vi "AddTestSuite.vi"(8 "error in (no error)":errorcluster, 9 "Name":string, 10 "Parent Tag (\"\")":string, 11 "ResultTree in":refnum<class "ResultTree.lvclass">) -> (0 "error out":errorcluster, 2 "Tag Name":string, 3 "ResultTree out":refnum<class "ResultTree.lvclass">)   [LabVIEW 2017, in "ResultTree.lvclass"]
doc: "Adds a test suite. Returns the tag name.\n\nIf no parent tag is specified, the test suite is added to the root and tagged with the prefix \"SUITE_\" followed by the name of the suite.\n\nIf a parent tag is specified, the test suite is added as a child to the parent suite with the parent suite name as prefix followed by \"/\" and the name of the suite."
uses:
  ResultTree.lvclass
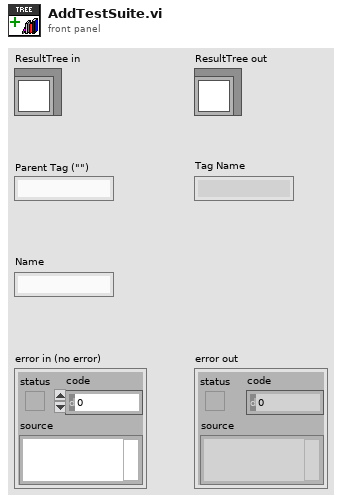
[diagram p1: front panel]
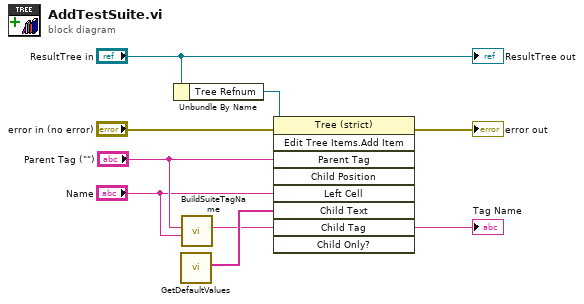
[diagram p0: block diagram]
diagram:
  n1 = Unbundle By Name("ResultTree in") -> ("Tree Refnum"=w5:refnum<vi>)
  n2 = call "GetDefaultValues.vi"() -> ("Default Values"=w4:string[])  [unwired: 11 in]
  n3 = call "BuildSuiteTagName.vi"("Suite Name"="Name", "Parent Tag"="Parent Tag (\"\")") -> ("Tag Name"=w1:string)  [unwired: 9 in]
  "Tag Name" <- w1
  n4 = invoke class="Tree (strict)" method="Edit Tree Items.Add Item"(reference=w5, error in="error in (no error)", "Parent Tag"="Parent Tag (\"\")", "Left Cell"="Name", "Child Text"=w4, "Child Tag"=w1) -> (error out=→"error out":errorcluster)  [unwired: 3 in, 8 out]
  "ResultTree out" <- "ResultTree in"
